vi "sabertooth packetized v2.vi"() -> ()   [LabVIEW 2018]
uses:
  <vilib>/myRIO/Instrument Drivers/Onboard IO/UART/typedef/VISA Configuration.ctl
  <vilib>/Instr/_visa.llb/VISA Configure Serial Port (Instr).vi
  <vilib>/myRIO/Instrument Drivers/Onboard IO/UART/UART.lvlib
panel:
  out "x-y":u32
  in  "Motor Speed 4":dbl(knob) scale=-1.0..1.0
  in  "Motor Speed 3":dbl(knob) scale=-1.0..1.0
  in  "Motor Speed 2":dbl(knob) scale=-1.0..1.0
  in  "Motor Speed 1":dbl(knob) scale=-1.0..1.0
  in  "stop":bool
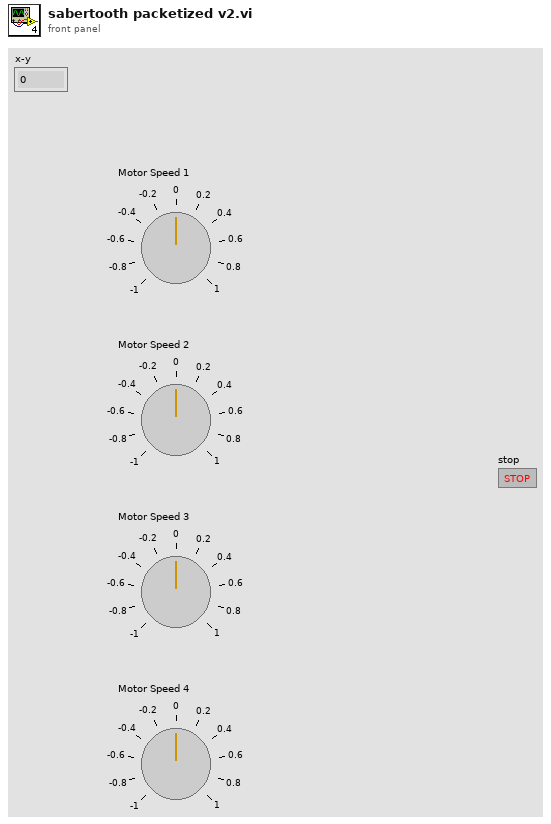
[diagram p1: front panel]
types:
  T1 = typedef "UART.lvlib/VISA Configuration.ctl" = cluster{"baud rate (9600)":u32, "data bits (8)":u16, "parity (0:none)":enum16{"None", "Odd", "Even", "Mark", "Space"}, "stop bits (10: 1 bit)":u16, "flow control (0:none)":u16, "termination char\n(0xA = '\\n' = LF) ":u8, "Enable Termination\nChar (T)":bool, "timeout (10sec)":u32}
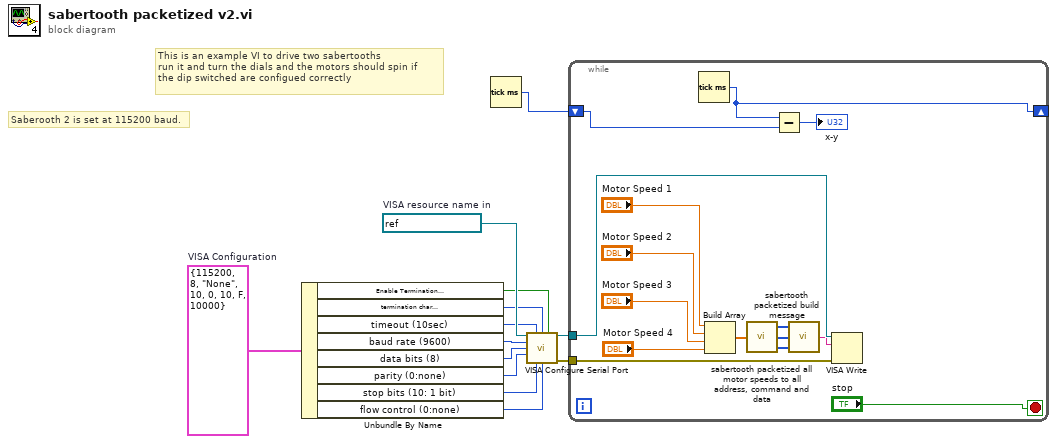
[diagram p0: block diagram]
diagram:
  w12 = T1 {"baud rate (9600)"=115200, "data bits (8)"=8, "parity (0:none)"=enum."None", "stop bits (10: 1 bit)"=10, "flow control (0:none)"=0, "termination char\n(0xA = '\\n' = LF) "=10, "Enable Termination\nChar (T)"=FALSE, "timeout (10sec)"=10000}  # VISA Configuration
  w13 = refnum<visa-resource-name> "ASRL1::INSTR"  # VISA resource name in
  # "Saberooth 2 is set at 115200 baud."
  # "This is an example VI to drive two sabertooths\nrun it and turn the dials and the motors should spin if \nthe dip switched are configued correctly"
  n1 = Unbundle By Name(w12) -> ("Enable Termination\nChar (T)"=w9:bool, "termination char\n(0xA = '\\n' = LF)"=w8:u8, "timeout (10sec)"=w7:u32, "baud rate (9600)"=w2:u32, "data bits (8)"=w3:u16, "parity (0:none)"=w4:enum16{"None", "Odd", "Even", "Mark", "Space"}, "stop bits (10: 1 bit)"=w5:u16, "flow control (0:none)"=w6:u16)
  n2 = Tick Count (ms)() -> (millisecond timer value=w1:u32)
  n3 = call-poly "VISA Configure Serial Port"("VISA resource name"=w13, "timeout (10sec)"=w7, "termination char\n(0xA = '\\n' = LF)"=w8, "Enable Termination\nChar (T)"=w9, "baud rate (9600)"=w2, "data bits (8)"=w3, "parity (0:none)"=w4, "stop bits (10: 1 bit)"=w5, "flow control (0:none)"=w6) -> ("VISA resource name out"=w11:refnum<visa-resource-name>, "error out"=w10:errorcluster)  [unwired: 5 in]
  n4 = while {
    tunnel: w11 -> [w28]
    tunnel: w10 -> [w26]
    shift-right: [w14] -> _
    shift-left: w1 -> [w16]
    stop <- "stop" stop-if-true
    n5 = Tick Count (ms)() -> (millisecond timer value=w14:u32)
    n6 = Build Array("Motor Speed 1", "Motor Speed 2", "Motor Speed 3", "Motor Speed 4") -> (w17:dbl[])
    n7 = call "sabertooth packetized all motor speeds to all address, command and data.vi"("All Motor Speeds"=w17) -> ("All Addresses"=w25:u8[], "All Commands"=w24:u8[], "All Data"=w23:u8[])
    n8 = Subtract(x=w14, y=w16) -> (x-y=→"x-y":u32)
    n9 = call "sabertooth packetized build message.vi"("All Data"=w23, "All Commands"=w24, "All Addresses"=w25) -> ("Uart Write Data"=w22:string)
    n10 = VISA Write(VISA resource name=w28, write buffer=w22, error in (no error)=w26) -> ()  [unwired: 3 out]
  }
